vi "Start Streaming.vi"(8 "error in (no error)":errorcluster, 9 "Camera Settings":T1={"Exposure Time (ms)"=100.0, "Binning"=enum."2x2", "Scan Mode"=-1, "Frames to Acquire"=1000.0, "Pixel Correction"=FALSE, "Frames to Skip"=1, "File Path"=path "", "Duty cycle"=1.0, "ALEX"=FALSE, "Shutter Enable"=[], "fluidics trigger, ms (0=disabled)"=0.0, "Bit Depth"=16, "Image Width (px)"=0, "Image Height (px)"=0, "Horizontal Offset (px)"=0, "Vertical Offset (px)"=0} {"fluidics trigger, ms (0=disabled)" max=60000.0 step=1.0; "Exposure Time (ms)" min=1.0 max=10000.0 step=1.0}, 11 "Synchronization Device in":refnum<class "Microsync.lvclass">) -> (0 "error out":errorcluster, 3 "Synchronization Device out":refnum<class "Microsync.lvclass">)   [LabVIEW 2023, in "Microsync.lvlib" / "Microsync.lvclass"]
uses:
  Microsync.lvclass
  Resources/Type Defs/Camera Settings.ctl
  Microsync.lvclass/Microsync.ctl
  34cc9672-883f-4aa2-b08b-d0e88a6c2352.vi
  Resources/GLOBAL/GLOBAL Time-critical.vi
  Sync Device/Sync Device.lvclass
  Microsync.lvlib
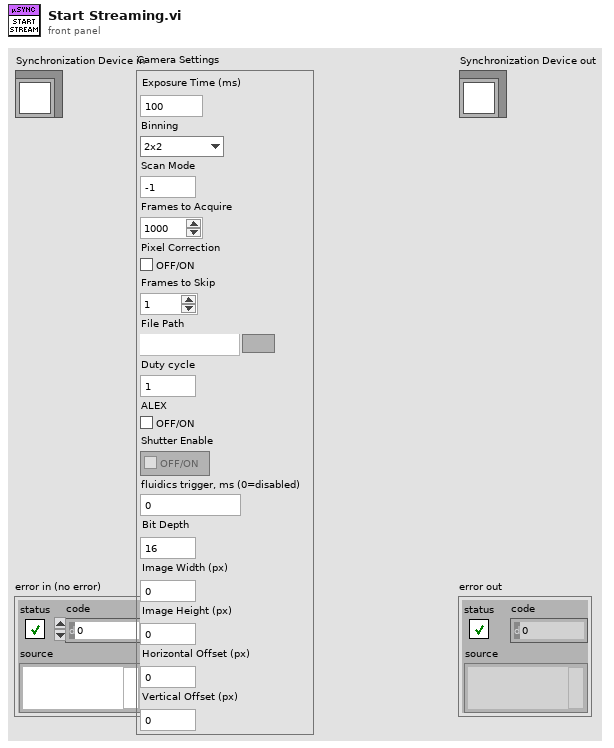
[diagram p1: front panel]
types:
  T1 = typedef "Camera Settings.ctl" = cluster{"Exposure Time (ms)":dbl, "Binning":enum16{"1x1", "2x2", "4x4"}, "Scan Mode":i32, "Frames to Acquire":dbl, "Pixel Correction":bool, "Frames to Skip":u32, "File Path":path, "Duty cycle":dbl, "ALEX":bool, "Shutter Enable":bool[], "fluidics trigger, ms (0=disabled)":dbl, "Bit Depth":u16, "Image Width (px)":u16, "Image Height (px)":u16, "Horizontal Offset (px)":u16, "Vertical Offset (px)":u16}
  T2 = enum16{"ro_VERSION", "ro_SYS_TIMER_STATUS", "ro_SYS_TIMER_VALUE", "ro_SYS_TIMER_OVF_COUNT", "ro_SYS_TIME_ms", "ro_SYS_TIMER_PRESCALER", "rw_DFLT_PULSE_DURATION_us", "ro_WATCHDOG_TIMEOUT_ms", "ro_N_EVENTS", "rw_INTLCK_ENABLED", "rw_SELECTED_LASERS", "wo_OPEN_SHUTTERS", "wo_CLOSE_SHUTTERS", "rw_SHUTTER_DELAY_us", "rw_CAM_READOUT_us"}
  T3 = cluster{"interval_us":u32, "N":u32, "timestamp_us":u32, "arg2":u32, "arg1":u32}
  T4 = cluster{"interval_us":u32, "N":u32, "timestamp_us":u32, "arg2":u32, "Pin":string}
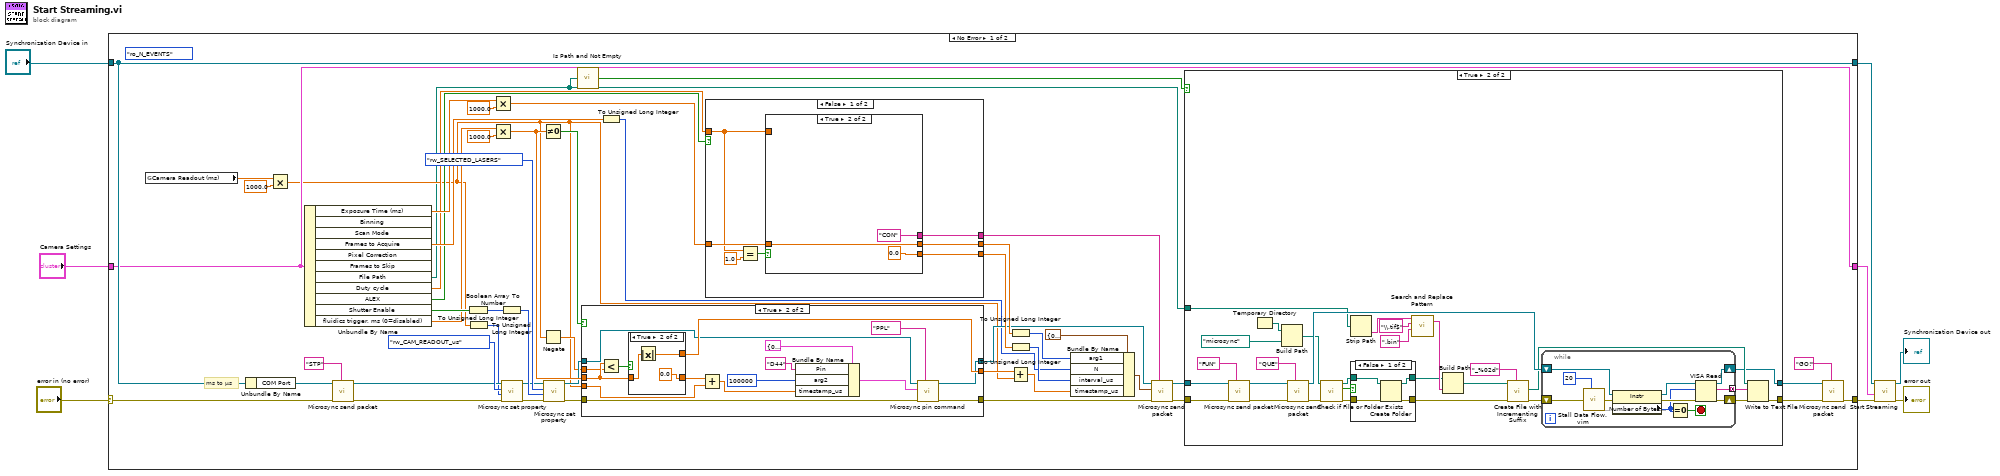
[diagram p0: block diagram]
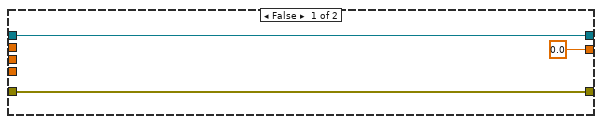
[diagram p4: hidden frame]
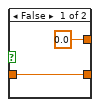
[diagram p5: hidden frame]
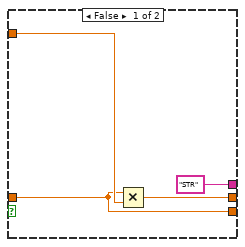
[diagram p6: hidden frame]
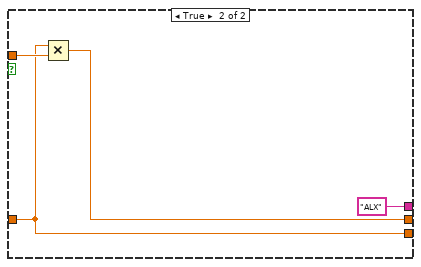
[diagram p7: hidden frame]
diagram:
  n1 = case shown="No Error" "error in (no error)" {
    selector: "error in (no error)" -> [w45 w152]
    tunnel: [w30 w152] -> w5
    tunnel: [w59 w151] -> w4
    tunnel: "Synchronization Device in" -> [w59 w151]
    tunnel: "Camera Settings" -> [w43 w150]
    tunnel: [w43 w150] -> w1
    frame No Error {
      (unwired) T2."ro_N_EVENTS" ("Property to get")
      # "ms to µs"
      n2 = global read "GLOBAL Time-critical.vi" "Camera Readout (ms)"() -> (w37:dbl)
      n3 = Unbundle By Name(w59) -> ("COM Port"=w44:refnum<visa-resource-name>)
      n4 = Multiply(x=w37, y=1000.0) -> (x*y=w16:dbl)
      n5 = Unbundle By Name(w43) -> ("Exposure Time (ms)"=w58:dbl, "Frames to Acquire"=w55:dbl, "File Path"=w9:path, "Duty cycle"=w52:dbl, "ALEX"=w54:bool, "Shutter Enable"=w40:bool[], "fluidics trigger, ms (0=disabled)"=w27:dbl)  [unwired: 4 out]
      n6 = call "Microsync send packet.vi"("Command"="STP", "error in (no error)"=w45, "VISA resource name"=w44) -> ("error out"=w34:errorcluster, "VISA resource name out"=w35:refnum<visa-resource-name>)  [unwired: 6 in, 1 out]
      n7 = Boolean Array To Number(Boolean array=w40) -> (number=w41:u32)
      n8 = To Unsigned Long Integer(number=w16) -> (unsigned 32bit integer=w18:u32)
      n9 = Multiply(x=w58, y=1000.0) -> (x*y=w49:dbl)
      n10 = Multiply(x=w27, y=1000.0) -> (x*y=w26:dbl)
      n11 = To Unsigned Long Integer(number=w41) -> (unsigned 32bit integer=w39:u32)
      n12 = call "Microsync set property.vi"("error in (no error)"=w34, "Property value"=w18, "property to set"=T2."rw_CAM_READOUT_us", "VISA resource name"=w35) -> ("error out"=w32:errorcluster, "VISA resource name out"=w33:refnum<visa-resource-name>)  [unwired: 6 in]
      n13 = Not Equal To 0?(x=w26) -> (x != 0?=w21:bool)
      n14 = Negate(x=w16) -> (-x=w17:dbl)
      n15 = call "Microsync set property.vi"("error in (no error)"=w32, "Property value"=w39, "property to set"=T2."rw_SELECTED_LASERS", "VISA resource name"=w33) -> ("error out"=w24:errorcluster, "VISA resource name out"=w25:refnum<visa-resource-name>)  [unwired: 6 in]
      n16 = call <vilib>:"Is Path and Not Empty.vi"("path"=w9) -> ("Is Path and Not Empty?"=w14:bool)  [unwired: 4 in]
      n17 = case shown="True" w21 {
        tunnel: [0.0 w121] -> w19
        tunnel: w26 -> [_ w113]
        tunnel: w25 -> [w110 w120]
        tunnel: w24 -> [w109 w119]
        tunnel: [w110 w118] -> w23
        tunnel: [w109 w117] -> w22
        tunnel: w16 -> [_ w115]
        tunnel: w17 -> [_ w112]
        frame False {
        }
        frame True {
          n18 = Less?(x=w113, y=w112) -> (x < y?=w111:bool)
          n19 = case shown="True" w111 {
            tunnel: w113 -> [w127 w130]
            tunnel: [0.0 w129] -> w121
            tunnel: [w127 0.0] -> w116
            frame False {
            }
            frame True {
              n20 = Absolute Value(x=w130) -> (abs(x)=w129:dbl)
            }
          }
          n21 = Add(x=w116, y=w115) -> (x+y=w114:dbl)
          n22 = Bundle By Name(cluster=T4 {"interval_us"=0, "N"=0, "timestamp_us"=0, "arg2"=0, "Pin"=""} ("Arguments"), "Pin"="D44", "arg2"=u32 100000, "timestamp_us"=w114) -> (w123:T4)
          n23 = call "Microsync pin command.vi"("Combo Box"="PPL", "error in (no error)"=w119, "Arguments"=w123, "VISA resource name"=w120) -> ("error out"=w117:errorcluster, "VISA resource name out"=w118:refnum<visa-resource-name>)  [unwired: 5 in, 1 out]
        }
      }
      n24 = To Unsigned Long Integer(number=w55) -> (unsigned 32bit integer=w15:u32)
      n25 = case shown="False" w54 {
        tunnel: [w138 "ALX" ("Command")] -> w53
        tunnel: w52 -> [w134 w148]
        tunnel: w49 -> [w136 w146]
        tunnel: [w135 w147] -> w51
        tunnel: [w133 w146] -> w47
        frame False {
          n26 = Equal?(x=w134, y=1.0) -> (x = y?=w137:bool)
          n27 = case shown="True" w137 {
            tunnel: ["STR" ("Command") "CON" ("Command")] -> w138
            tunnel: w136 -> [w139 w144]
            tunnel: [w140 w144] -> w135
            tunnel: w134 -> [w141 _]
            tunnel: [w139 0.0] -> w133
            frame False {
              n28 = Multiply(x=w139, y=w141) -> (x*y=w140:dbl)
            }
            frame True {
            }
          }
        }
        frame True {
          n29 = Multiply(x=w146, y=w148) -> (x*y=w147:dbl)
        }
      }
      n30 = To Unsigned Long Integer(number=w51) -> (unsigned 32bit integer=w50:u32)
      n31 = To Unsigned Long Integer(number=w47) -> (unsigned 32bit integer=w48:u32)
      n32 = Add(x=w19, y=w16) -> (x+y=w20:dbl)
      n33 = Bundle By Name(cluster=T3 {"interval_us"=0, "N"=500, "timestamp_us"=0, "arg2"=0, "arg1"=127} ("Arguments"), "arg1"=w50, "N"=w15, "interval_us"=w48, "timestamp_us"=w20) -> (w56:T3)
      n34 = call "Microsync send packet.vi"("Command"=w53, "error in (no error)"=w22, "Arguments"=w56, "VISA resource name"=w23) -> ("error out"=w13:errorcluster, "VISA resource name out"=w12:refnum<visa-resource-name>)  [unwired: 5 in, 1 out]
      n35 = case shown="True" w14 {
        tunnel: w13 -> [w60 w71]
        tunnel: w12 -> [w61 w70]
        tunnel: [w61 w64] -> w11
        tunnel: [w60 w63] -> w10
        tunnel: w9 -> [_ w62]
        frame False {
        }
        frame True {
          n36 = call "Microsync send packet.vi"("Command"="FUN", "error in (no error)"=w71, "VISA resource name"=w70) -> ("error out"=w85:errorcluster, "VISA resource name out"=w84:refnum<visa-resource-name>)  [unwired: 6 in, 1 out]
          n37 = Temporary Directory() -> (w81:path)
          n38 = Build Path(base path=w81, name or relative path=path "microsync") -> (appended path=w78:path)
          n39 = call "Microsync send packet.vi"("Command"="QUE", "error in (no error)"=w85, "VISA resource name"=w84) -> ("error out"=w77:errorcluster, "VISA resource name out"=w87:refnum<visa-resource-name>)  [unwired: 6 in, 1 out]
          n40 = call <vilib>:"Check if File or Folder Exists.vi"("error in (no error)"=w77, "path"=w78) -> ("error out"=w73:errorcluster, "file or folder exists?"=w76:bool, "dup path"=w74:path)  [unwired: 7 in]
          n41 = Strip Path(path=w62) -> (name=w82:string)  [unwired: 1 out]
          n42 = case shown="False" w76 {
            tunnel: w73 -> [w105 w107]
            tunnel: w74 -> [w104 w106]
            tunnel: [w103 w107] -> w75
            tunnel: [w102 w106] -> w79
            frame False {
              n43 = Create Folder(path (use dialog)=w104, error in=w105) -> (created path=w102:path, error out=w103:errorcluster)  [unwired: 1 in, 1 out]
            }
            frame True {
            }
          }
          n44 = call <vilib>:"Search and Replace Pattern.vi"("string"=w82, "regular expression (\"\")"="\\.tif$" ("regular expression (\"\")"), "replace string (\"\")"=".bin" ("replace string (\"\")")) -> ("result string"=w83:string)  [unwired: 2 in, 1 out]
          n45 = Build Path(base path=w79, name or relative path=w83) -> (appended path=w80:path)
          n46 = call <vilib>:"Create File with Incrementing Suffix.vi"("format string (\" (%d)\")"="_%02d" ("format string (\" (%d)\")"), "error in (no error)"=w75, "file path"=w80) -> ("error out"=w88:errorcluster, "actual path"=w86:path)  [unwired: 6 in, 1 out]
          n47 = while {
            shift-right: [w92] -> w89
            shift-left: w88 -> [w94]
            shift-right: [w101] -> w64
            shift-left: w87 -> [w99]
            tunnel: [w100] -> w90 mode=concatenating
            stop <- w97 stop-if-true
            n48 = call "Stall Data Flow.vim"("value in"=w94, "milliseconds to wait"=u32 20) -> ("value out"=w93:errorcluster)  [unwired: 1 out]
            n49 = property class="Instr"(reference=w99, error in=w93) -> (reference out=w98:refnum<visa-resource-name>, error out=w96:errorcluster, "Serial Settings:Number of Bytes at Serial Port"=w91:u32)
            n50 = Equal To 0?(x=w91) -> (x = 0?=w97:bool)
            n51 = VISA Read(VISA resource name=w98, byte count=w91, error in (no error)=w96) -> (VISA resource name out=w101:refnum<visa-resource-name>, read buffer=w100:string, error out=w92:errorcluster)  [unwired: 1 out]
          }
          n52 = Write to Text File(file (use dialog)=w86, text=w90, error in=w89) -> (error out=w63:errorcluster)  [unwired: 1 in, 2 out]
        }
      }
      n53 = call "Microsync send packet.vi"("Command"="GO!", "error in (no error)"=w10, "VISA resource name"=w11) -> ("error out"=w30:errorcluster)  [unwired: 6 in, 2 out]
    }
    frame Error {
    }
  }
  n54 = call-parent "Start Streaming.vi"("error in (no error)"=w5, "Camera Settings"=w1, "Synchronization Device in"=w4) -> ("error out"=→"error out":errorcluster, "Synchronization Device out"=→"Synchronization Device out":refnum<class "Microsync.lvclass">)  [unwired: 7 in]
